vi "2283_seleccionDeNivel.vi"(5 "Nivel step":bool, 7 "Nivel 3 cajas":bool, 9 "Nivel 2 cajas":bool, 11 "Nivel 1 caja":bool, 13 "Nivel cargar":bool, 18 "Dejar":bool, 19 "Nivel piso":bool) -> (10 "nivel":T1(ring))   [LabVIEW 2014]
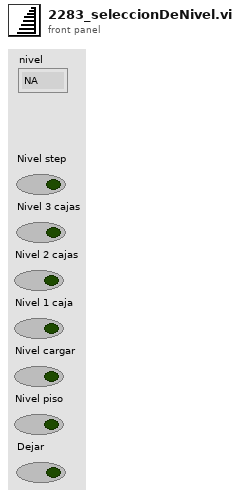
[diagram p1: front panel]
types:
  T1 = enum16{"NA", "Nivel cargar", "Nivel Techo", "Nivel step", "Nivel 3 cajas", "Nivel 2 cajas", "Nivel 1 caja", "Nivel Piso"}
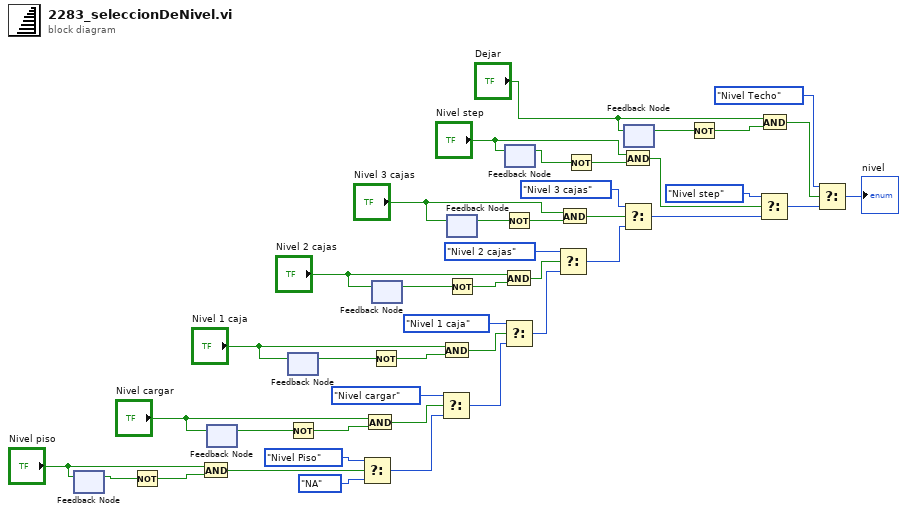
[diagram p0: block diagram]
diagram:
  n1 = feedback #1() -> (w14:bool)  [unwired: 1 in]
  n2 = feedback-in #1("Nivel piso") -> ()
  n3 = Not(x=w14) -> (.not. x?=w15:bool)
  n4 = And(x="Nivel piso", y=w15) -> (x .and. y?=w12:bool)
  n5 = feedback #2() -> (w18:bool)  [unwired: 1 in]
  n6 = feedback-in #2("Nivel cargar") -> ()
  n7 = feedback #3() -> (w22:bool)  [unwired: 1 in]
  n8 = feedback-in #3("Nivel 1 caja") -> ()
  n9 = Not(x=w18) -> (.not. x?=w19:bool)
  n10 = Select(t=T1."Nivel Piso" ("Enum"), s=w12, f=T1."NA" ("Enum")) -> (s? t:f=w11:T1)
  n11 = And(x="Nivel cargar", y=w19) -> (x .and. y?=w17:bool)
  n12 = Not(x=w22) -> (.not. x?=w23:bool)
  n13 = feedback #4() -> (w26:bool)  [unwired: 1 in]
  n14 = feedback-in #4("Nivel 2 cajas") -> ()
  n15 = Select(t=T1."Nivel cargar" ("Enum"), s=w17, f=w11) -> (s? t:f=w39:T1)
  n16 = And(x="Nivel 1 caja", y=w23) -> (x .and. y?=w20:bool)
  n17 = feedback #5() -> (w30:bool)  [unwired: 1 in]
  n18 = feedback-in #5("Nivel 3 cajas") -> ()
  n19 = Not(x=w26) -> (.not. x?=w27:bool)
  n20 = Not(x=w30) -> (.not. x?=w31:bool)
  n21 = And(x="Nivel 2 cajas", y=w27) -> (x .and. y?=w24:bool)
  n22 = Select(t=T1."Nivel 1 caja" ("Enum"), s=w20, f=w39) -> (s? t:f=w40:T1)
  n23 = feedback #6() -> (w34:bool)  [unwired: 1 in]
  n24 = feedback-in #6("Nivel step") -> ()
  n25 = Select(t=T1."Nivel 2 cajas" ("Enum"), s=w24, f=w40) -> (s? t:f=w41:T1)
  n26 = And(x="Nivel 3 cajas", y=w31) -> (x .and. y?=w28:bool)
  n27 = Not(x=w34) -> (.not. x?=w35:bool)
  n28 = And(x="Nivel step", y=w35) -> (x .and. y?=w32:bool)
  n29 = Select(t=T1."Nivel 3 cajas" ("Enum"), s=w28, f=w41) -> (s? t:f=w42:T1)
  n30 = feedback #7() -> (w37:bool)  [unwired: 1 in]
  n31 = feedback-in #7("Dejar") -> ()
  n32 = Not(x=w37) -> (.not. x?=w38:bool)
  n33 = Select(t=T1."Nivel step" ("Enum"), s=w32, f=w42) -> (s? t:f=w43:T1)
  n34 = And(x="Dejar", y=w38) -> (x .and. y?=w36:bool)
  n35 = Select(t=T1."Nivel Techo" ("Enum"), s=w36, f=w43) -> (s? t:f=→"nivel":T1)
